vi "Lithography Legacy Convert_Cypher.vi"(1 "Amplifier Setting":dbl=-15.0, 2 "Lithography Data":T2(array[cluster])) -> (0 "Array":T3(array[cluster]))   [LabVIEW 2019]
uses:
  <userlib>/LevyLab/Relay Box/Typedefs/Resistor--enum.ctl
  <userlib>/LevyLab/Relay Box/Relay-Box.lvclass
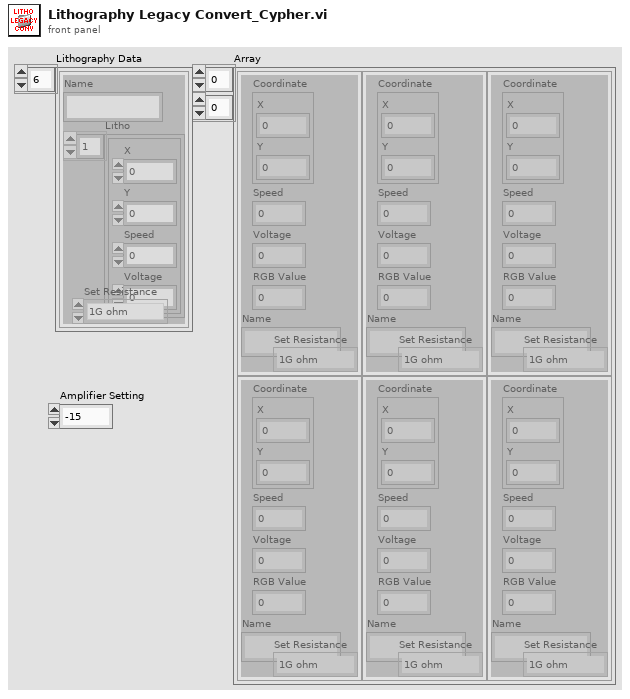
[diagram p1: front panel]
types:
  T1 = typedef "Relay-Box.lvclass/Resistor--enum.ctl" = enum16{"open", "discharge tip", "0 ohms", "100k ohm", "10M ohm", "1G ohm"}
  T2 = cluster{"Name":string, "Litho":cluster{"X":dbl, "Y":dbl, "Speed":dbl, "Voltage":dbl}[], "Set Resistance":T1}[]
  T3 = cluster{"Coordinate":cluster{"X":dbl, "Y":dbl}, "Speed":dbl, "Voltage":dbl, "RGB Value":dbl, "Name":string, "Set Resistance":T1}[][]
  T4 = cluster{"Coordinate":cluster{"X":dbl, "Y":dbl}, "Speed":dbl, dbl, "Voltage":dbl, "Name":string, "Set Resistance":T1}[][]
  T5 = cluster{"X":dbl, "Y":dbl, "Speed":dbl, "Voltage":dbl}[]
  T6 = cluster{"Coordinate":cluster{"X":dbl, "Y":dbl}, "Speed":dbl, dbl, "Voltage":dbl, "Name":string, "Set Resistance":T1}
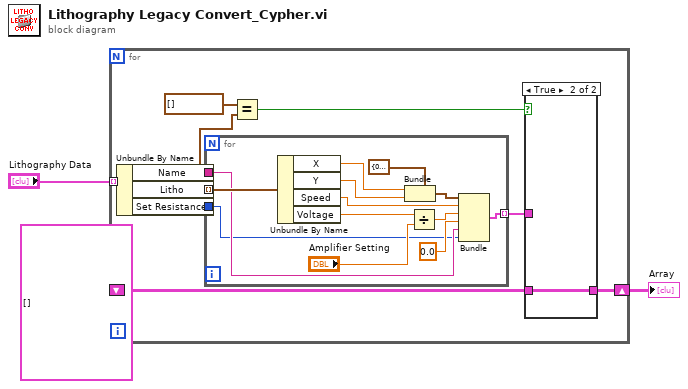
[diagram p0: block diagram]
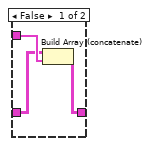
[diagram p2: hidden frame]
diagram:
  n1 = for {
    tunnel: "Lithography Data" -> [w12] mode=indexing
    shift-right: [w10] -> w1
    shift-left: T4 [] -> [w9]
    n2 = Unbundle By Name(w12) -> ("Name"=w11:string, "Litho"=w5:T5, "Set Resistance"=w4:T1)
    n3 = for {
      tunnel: w5 -> [w29] mode=indexing
      tunnel: w11 -> [w23]
      tunnel: [w22] -> w8 mode=indexing
      tunnel: w4 -> [w17]
      n4 = Unbundle By Name(w29) -> ("X"=w28:dbl, "Y"=w27:dbl, "Speed"=w24:dbl, "Voltage"=w20:dbl)
      n5 = Bundle(cluster=cluster{"X":dbl, "Y":dbl} {"X"=0.0, "Y"=0.0} ("Coordinate"), "X"=w28, "Y"=w27) -> (w25:cluster{"X":dbl, "Y":dbl})
      n6 = Divide(x=w20, y="Amplifier Setting") -> (x/y=w19:dbl)
      n7 = Bundle("Coordinate"=w25, "Speed"=w24, w19, "Voltage"=0.0, "Name"=w23, "Set Resistance"=w17) -> (w22:T6)  [unwired: 1 in]
    }
    n8 = Equal?(x=T5 [] ("Litho"), y=w5) -> (x = y?=w7:bool)
    n9 = case shown="True" w7 {
      tunnel: [w15 w16] -> w10
      tunnel: w9 -> [w13 w16]
      tunnel: w8 -> [w14 _]
      frame False {
        n10 = Build Array (concatenate)(w13, w14) -> (w15:T4)
      }
      frame True {
      }
    }
  }
  "Array" <- w1
